vi "_wmg_PNtoPNwhereConnect.vi"(1 "Input":string) -> (0 "Output":string)   [LabVIEW 2011]
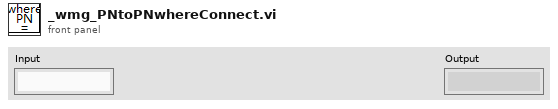
[diagram p1: front panel]
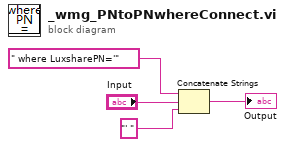
[diagram p0: block diagram]
diagram:
  n1 = Concatenate Strings(" where LuxsharePN='", "Input", "' ") -> (→"Output":string)
